vi "Read Write Digital Output.vi"(5 "Mode (F: Get)":bool, 7 "Unit Address (1)":i16=1, 8 "error in (no error)":errorcluster {"code" format="%.0x"}, 9 "Output Value (F: Off)":bool, 10 "Digital Output (1)":i16=1, 11 "VISA resource name":refnum<visa-resource-name>) -> (0 "error out":errorcluster {"code" format="%.0x"}, 2 "Output Value":bool, 3 "VISA resource name out":refnum<visa-resource-name>)   [LabVIEW 2010]
doc: "This VI is used to read or write Digital Output values."
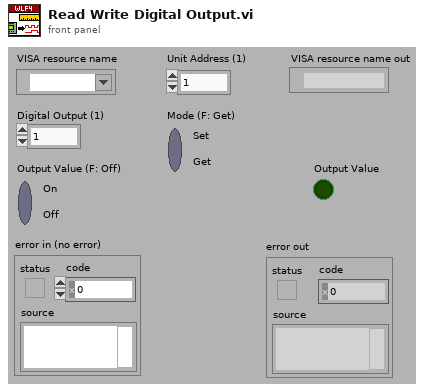
[diagram p1: front panel]
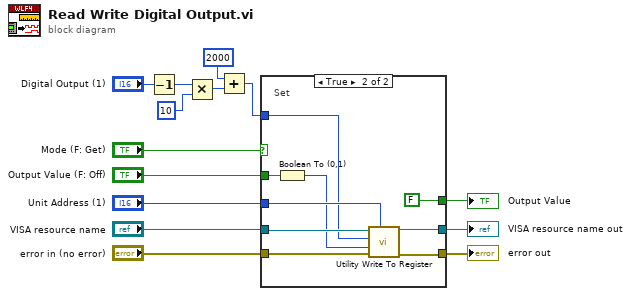
[diagram p0: block diagram]
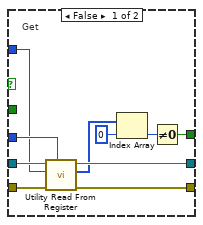
[diagram p2: hidden frame]
diagram:
  n1 = Decrement(x="Digital Output (1)") -> (x-1=w8:i16)
  n2 = Multiply(x=w8, y=i16 10) -> (x*y=w5:i16)
  n3 = Add(x=2000 ("index"), y=w5) -> (x+y=w4:i32)
  n4 = case shown="True" "Mode (F: Get)" {
    tunnel: "Unit Address (1)" -> [w24 w30]
    tunnel: "VISA resource name" -> [w23 w29]
    tunnel: "error in (no error)" -> [w22 w33]
    tunnel: [w21 w32] -> w11
    tunnel: [w20 w31] -> w10
    tunnel: w4 -> [w16 w28]
    tunnel: [w15 FALSE] -> w3
    tunnel: "Output Value (F: Off)" -> [_ w26]
    frame False {
      # "Get"
      n5 = call "Utility Read From Register.vi"("Unit Address (1)"=w24, "error in (no error)"=w22, "Register Address (0)"=w16, "VISA resource name"=w23) -> ("error out"=w21:errorcluster, "Data"=w18:i16[], "VISA resource name out"=w20:refnum<visa-resource-name>)  [unwired: 5 in]
      n6 = Index Array(array=w18, index=0) -> (element=w17:i16)
      n7 = Not Equal To 0?(x=w17) -> (x != 0?=w15:bool)
    }
    frame True {
      # "Set"
      n8 = Boolean To (0,1)(Boolean=w26) -> (0, 1=w25:i16)
      n9 = call "Utility Write To Register.vi"("Unit Address (1)"=w30, "error in (no error)"=w33, "Data (0)"=w25, "Register Address (0)"=w28, "VISA resource name"=w29) -> ("error out"=w32:errorcluster, "VISA resource name out"=w31:refnum<visa-resource-name>)  [unwired: 5 in]
    }
  }
  "error out" <- w11
  "VISA resource name out" <- w10
  "Output Value" <- w3
